vi "FTW-Regex.vi"(0 "Regular Expression":string, 5 "Input String":string, 7 "Include Empty Capture Groups (F)":bool, 9 "Starting Offset":i32, 11 "error in":errorcluster) -> (4 "Match":string, 6 "Submatches":string[](array[string]), 8 "Match Found?":bool, 10 "Offset after Match":i32, 15 "error out":errorcluster)   [LabVIEW 2015]
panel:
  out "Match Offsets":i32[](array[numeric])
  # "Inputs"
  # "Debug"
  # "Outputs"
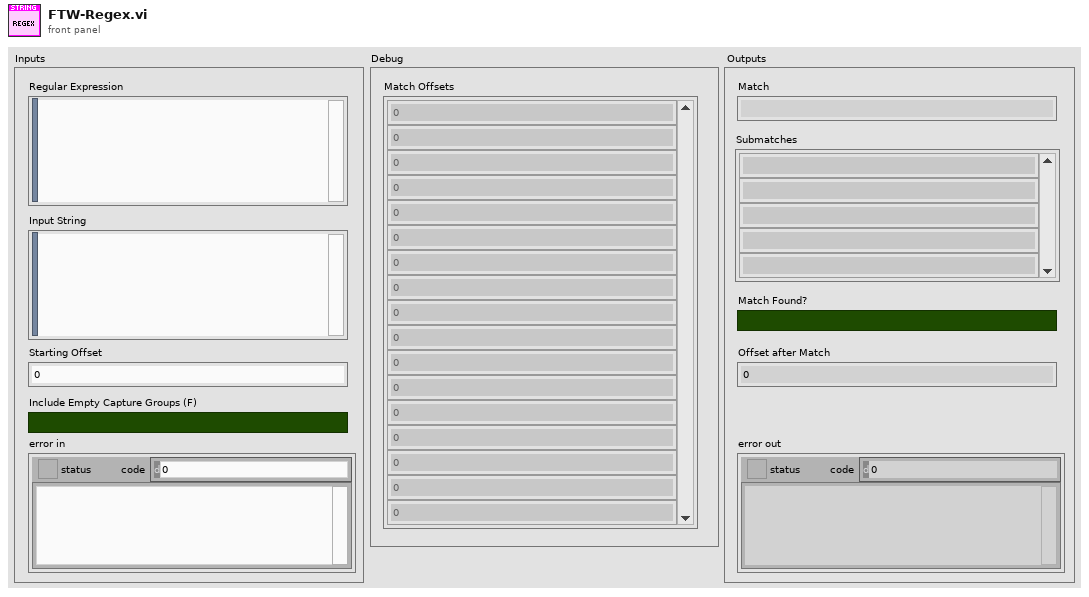
[diagram p1: front panel]
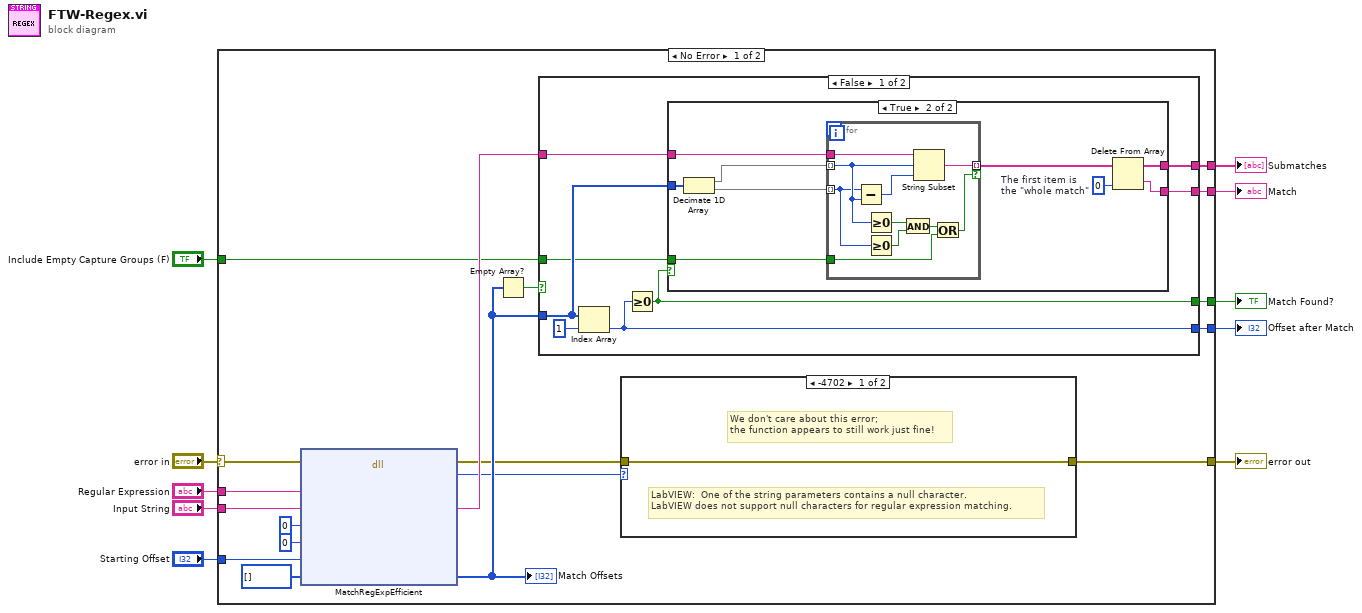
[diagram p0: block diagram]
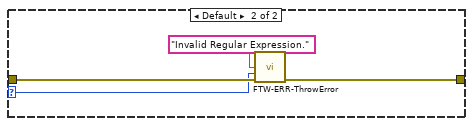
[diagram p2: hidden frame]
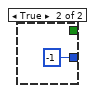
[diagram p4: hidden frame]
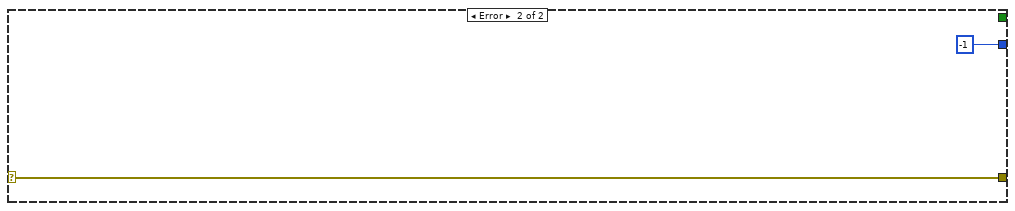
[diagram p5: hidden frame]
diagram:
  n1 = case shown="No Error" "error in" {
    selector: "error in" -> [w15 w62]
    tunnel: "Regular Expression" -> [w28 _]
    tunnel: [w27 _] -> w9
    tunnel: [w26 _] -> w8
    tunnel: [w13 w62] -> w7
    tunnel: "Starting Offset" -> [w25 _]
    tunnel: [w24 -1] -> w5
    tunnel: [w23 _] -> w4
    tunnel: "Input String" -> [w22 _]
    tunnel: "Include Empty Capture Groups (F)" -> [w11 _]
    frame No Error {
      n2 = dll-call lib="LabVIEW" fn="MatchRegExpEfficient"(error in=w15, "Regular Expression"=w28, "Subject"=w22, "Ignore Case?"=0, "Multiline?"=0, "Starting Offset"=w25, "Match Offsets"=i32[] []) -> (error out=w14:errorcluster, "Return"=w12:i32, "Subject"=w21:string, "Match Offsets"=w17:i32[])  [unwired: 6 in, 1 out]
      "Match Offsets" <- w17
      n3 = Empty Array?(array=w17) -> (empty?=w16:bool)
      n4 = case shown="False" w16 {
        tunnel: [w41 _] -> w27
        tunnel: [w40 _] -> w26
        tunnel: [w38 -1] -> w24
        tunnel: [w37 _] -> w23
        tunnel: w21 -> [w36 _]
        tunnel: w17 -> [w35 _]
        tunnel: w11 -> [w34 _]
        frame False {
          n5 = Index Array(array=w35, index=1) -> (element=w38:i32)
          n6 = Greater Or Equal To 0?(x=w38) -> (x >= 0?=w37:bool)
          n7 = case shown="True" w37 {
            tunnel: w36 -> [_ w50]
            tunnel: [_ w46] -> w41
            tunnel: [_ w45] -> w40
            tunnel: w35 -> [_ w43]
            tunnel: w34 -> [_ w42]
            frame False {
            }
            frame True {
              w47 = 0  # The first item is the "whole match"
              n8 = Decimate 1D Array(w43) -> (w49:i32[], w44:i32[])
              n9 = for {
                tunnel: w50 -> [w60]
                tunnel: [w59] -> w48 mode=indexing if=w52
                tunnel: w49 -> [w57] mode=indexing
                tunnel: w44 -> [w53] mode=indexing
                tunnel: w42 -> [w51]
                n10 = Subtract(x=w53, y=w57) -> (x-y=w58:i32)
                n11 = Greater Or Equal To 0?(x=w57) -> (x >= 0?=w56:bool)
                n12 = Greater Or Equal To 0?(x=w53) -> (x >= 0?=w55:bool)
                n13 = And(x=w56, y=w55) -> (x .and. y?=w54:bool)
                n14 = String Subset(string=w60, offset (0)=w57, length (rest)=w58) -> (substring=w59:string)
                n15 = Or(x=w54, y=w51) -> (x .or. y?=w52:bool)
              }
              n16 = Delete From Array(array=w48, index=w47) -> (deleted portion=w46:string, array with subset deleted=w45:string[])  [unwired: 1 in]
            }
          }
        }
        frame True {
        }
      }
      n17 = case shown="-4702" w12 {
        selector: w12 -> [_ w30]
        tunnel: w14 -> [w29 w33]
        tunnel: [w29 w32] -> w13
        frame -4702 {
          # "We don't care about this error;\nthe function appears to still work just fine!"
          # "LabVIEW:  One of the string parameters contains a null character.\nLabVIEW does not support null characters for regular expression matching."
        }
        frame Default {
          n18 = call "FTW-ERR-ThrowError.vi"("Error Message"="Invalid Regular Expression.", "Error Code"=w30, "error in"=w33) -> ("error out"=w32:errorcluster)  [unwired: 12 in]
        }
      }
    }
    frame Error {
    }
  }
  "error out" <- w7
  "Submatches" <- w8
  "Match" <- w9
  "Match Found?" <- w4
  "Offset after Match" <- w5
